vi "Out_On_F5xxx.vi"(0 "DriverConnect in":T1={"InterfaceType"=enum."VISA", "OpenedSession"="", "InterfaceSettings"={"Interface"=enum."RS232", "EOS 4 read"=enum."LF (\\n)", "EOS 4 write"=enum."LF (\\n)", "TMO, ms"=10000, "Sett"=variant(cluster{"Baud Rate":u32, "Data Bits":u16, "Parity":u16, "Stop Bits":u16, "Flow Control":u16, "Eho":bool} {"Baud Rate"=75, "Data Bits"=0, "Parity"=0, "Stop Bits"=0, "Flow Control"=0, "Eho"=FALSE})}}, 1 "Model":dbl, 3 "Output Signal Auto ON":bool, 11 "error in":T6, 12 "Error Code":T8, 13 "Driver Name":T7) -> (4 "DriverConnect out":T1={"InterfaceType"=enum."VISA", "OpenedSession"="", "InterfaceSettings"={"Interface"=enum."RS232", "EOS 4 read"=enum."LF (\\n)", "EOS 4 write"=enum."LF (\\n)", "TMO, ms"=10000, "Sett"=variant(cluster{"Baud Rate":u32, "Data Bits":u16, "Parity":u16, "Stop Bits":u16, "Flow Control":u16, "Eho":bool} {"Baud Rate"=75, "Data Bits"=0, "Parity"=0, "Stop Bits"=0, "Flow Control"=0, "Eho"=FALSE})}}, 15 "error out":T6)   [LabVIEW 2018]
uses:
  MOKO_LabViewLibrary/MokoLowLevel/MokoLowLovelControl/MLLC_ErrorCode.ctl
  MOKO_LabViewLibrary/MokoLowLevel/MokoLowLovelControl/MLLC_DriverName.ctl
  MOKO_LabViewLibrary/MokoLowLevel/MokoLowLovelControl/MLLC_Error.ctl
  MOKO_LabViewLibrary/MokoLowLevel/MokoLowLovelControl/MLLC_ConnectCluster.ctl
  MOKO_LabViewLibrary/MokoLowLevel/MokoLowLovelControl/MLLC_InterfaceType.ctl
  MOKO_LabViewLibrary/MokoLowLevel/MokoLowLovelControl/MLLC_OpenedSession.ctl
  MOKO_LabViewLibrary/MokoLowLevel/MokoLowLovelControl/MLLC_InterfaceSettings.ctl
  MOKO_LabViewLibrary/MokoLowLevel/MokoLowLovelControl/MLLC_InterfaceKind.ctl
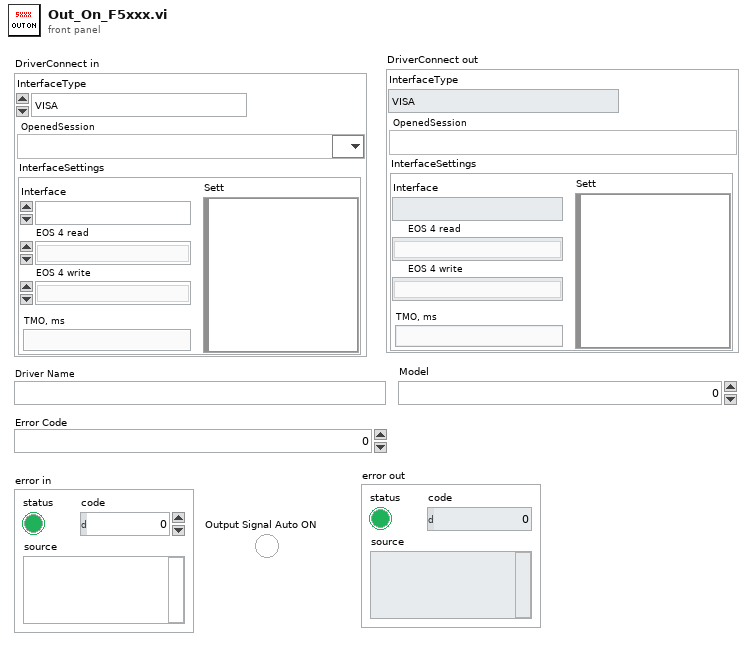
[diagram p1: front panel]
types:
  T1 = typedef "MLLC_ConnectCluster.ctl" = cluster{"InterfaceType":T2, "OpenedSession":T3, "InterfaceSettings":T4}
  T2 = typedef "MLLC_InterfaceType.ctl" = enum16{"VISA", "Prologix USB-GPIB"}
  T3 = typedef "MLLC_OpenedSession.ctl" = refnum<visa-resource-name>
  T4 = typedef "MLLC_InterfaceSettings.ctl" = cluster{"Interface":T5, "EOS 4 read":enum16{"Default (=EOS 4 write)", "CR (\\r)", "LF (\\n)", "None"}, "EOS 4 write":enum16{"CR+LF (\\r\\n)", "CR (\\r)", "LF (\\n)", "None"}, "TMO, ms":i32, "Sett":variant}
  T5 = typedef "MLLC_InterfaceKind.ctl" = enum16{"RS232", "GPIB", "USB", "Ethernet", "another"}
  T6 = typedef "MLLC_Error.ctl" = errorcluster
  T7 = typedef "MLLC_DriverName.ctl" = string
  T8 = typedef "MLLC_ErrorCode.ctl" = u32
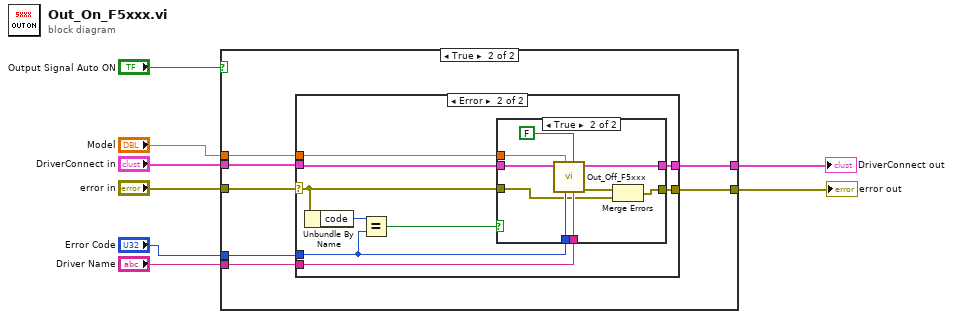
[diagram p0: block diagram]
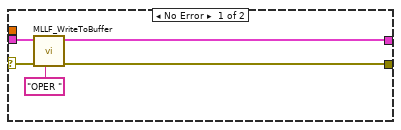
[diagram p3: hidden frame]
diagram:
  n1 = case shown="True" "Output Signal Auto ON" {
    tunnel: "Error Code" -> [_ w17]
    tunnel: "Driver Name" -> [_ w16]
    tunnel: [w10 w15] -> w6
    tunnel: "Model" -> [_ w14]
    tunnel: "error in" -> [w10 w13]
    tunnel: "DriverConnect in" -> [w9 w12]
    tunnel: [w9 w11] -> w1
    frame False {
    }
    frame True {
      n2 = case shown="Error" w13 {
        selector: w13 -> [w20 w27]
        tunnel: w12 -> [w21 w28]
        tunnel: w17 -> [_ w25]
        tunnel: w16 -> [_ w24]
        tunnel: [w18 w30] -> w15
        tunnel: [w19 w29] -> w11
        tunnel: w14 -> [_ w26]
        frame No Error {
          n3 = call "MLLF_WriteToBuffer.vi"("String"="OPER ", "error in"=w20, "DriverConnect in"=w21) -> ("error out"=w18:T6, "DriverConnect out"=w19:T1)  [unwired: 5 in]
        }
        frame Error {
          n4 = Unbundle By Name(w27) -> ("code"=w31:i32)
          n5 = Equal?(x=w31, y=w25) -> (x = y?=w23:bool)
          n6 = case shown="True" w23 {
            tunnel: [w32 w35] -> w30
            tunnel: [w33 w42] -> w29
            tunnel: w28 -> [w33 w41]
            tunnel: w27 -> [w32 w34]
            tunnel: w26 -> [_ w40]
            tunnel: w25 -> [_ w38]
            tunnel: w24 -> [_ w37]
            frame False {
            }
            frame True {
              n7 = call "Out_Off_F5xxx.vi"("Driver Name"=w37, "SwitchOFF"=FALSE, "Error Code"=w38, "Model"=w40, "DriverConnect in"=w41) -> ("error out"=w36:T6, "DriverConnect out"=w42:T1)  [unwired: 5 in]
              n8 = Merge Errors(w36, w34) -> (w35:errorcluster)
            }
          }
        }
      }
    }
  }
  "error out" <- w6
  "DriverConnect out" <- w1
